vi "NXT Camera Test6.vi"() -> ()   [LabVIEW 2016]
uses:
  <vilib>/NXT/Block Support/NXT_InputPort.ctl
  <vilib>/NXT/Block Support/NXT_OutputPort.ctl
  <vilib>/NXT/NXTIO Xnodes/NXTIONodeSubVIs/NXTMoveMotors.vi
  <vilib>/NXT/NXTIO Xnodes/NXTIONodeSubVIs/NXTStopMotors.vi
  <vilib>/NXT/Dual Mode Library/Waits/Wait_Num.vi
  <vilib>/NXT/Subs/LVHSConnector.ctl
  <vilib>/NXT/NXTIO Xnodes/AddressXNode/NXTIOAddress.xnode
  <vilib>/NXT/NXTIO Xnodes/NXTIOXNode/NXTIO.xnode
  <vilib>/NXT/LegoClasses/BrickReference/BrickReference.lvclass
panel:
  out "Power":bool
  out "X Upper Left":u8
  out "X Lower Right":u8
  out "Y Lower Right":u8
  out "Y Upper Left":u8
  out "Count":u8
  out "Color":u8
  in  "Cluster":T1 {"Tracking Mode" items=["Disable Tracking", "Get First Object", "Get n th Object", "Enable Tracking", "Sort Objects  by size", "Sort Objects  by Colors", "Illumination on ", "Illumination Off", "Write Colormap", "Read Colormap", "Line tracking mode", "Object Tracking mode"]}
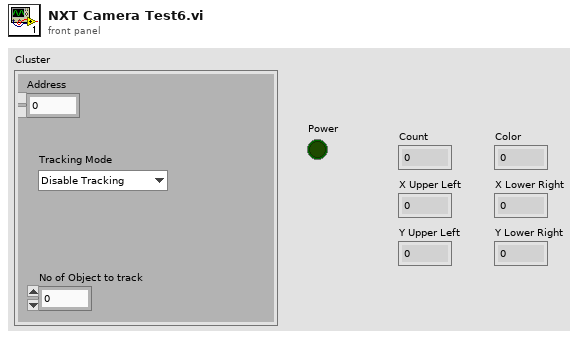
[diagram p1: front panel]
types:
  T1 = cluster{"Address":dbl, "No of Object to track":dbl, "Tracking Mode":u8}
  T2 = cluster{"Tracking Mode":u8, "Object Number to Track":u8, "Address":u8}
  T3 = typedef "NXT_InputPort.ctl" = u32
  T4 = typedef "LVHSConnector.ctl" = refnum<class "BrickReference.lvclass">
  T5 = cluster{"Total Tracked Objects":u8, "Color":u8, "X Upper Left":u8, "Y Upper Left":u8, "X Lower Right":u8, "Y Lower Right":u8, "Status (boolean)":bool}
  T6 = typedef "NXT_OutputPort.ctl" = u8
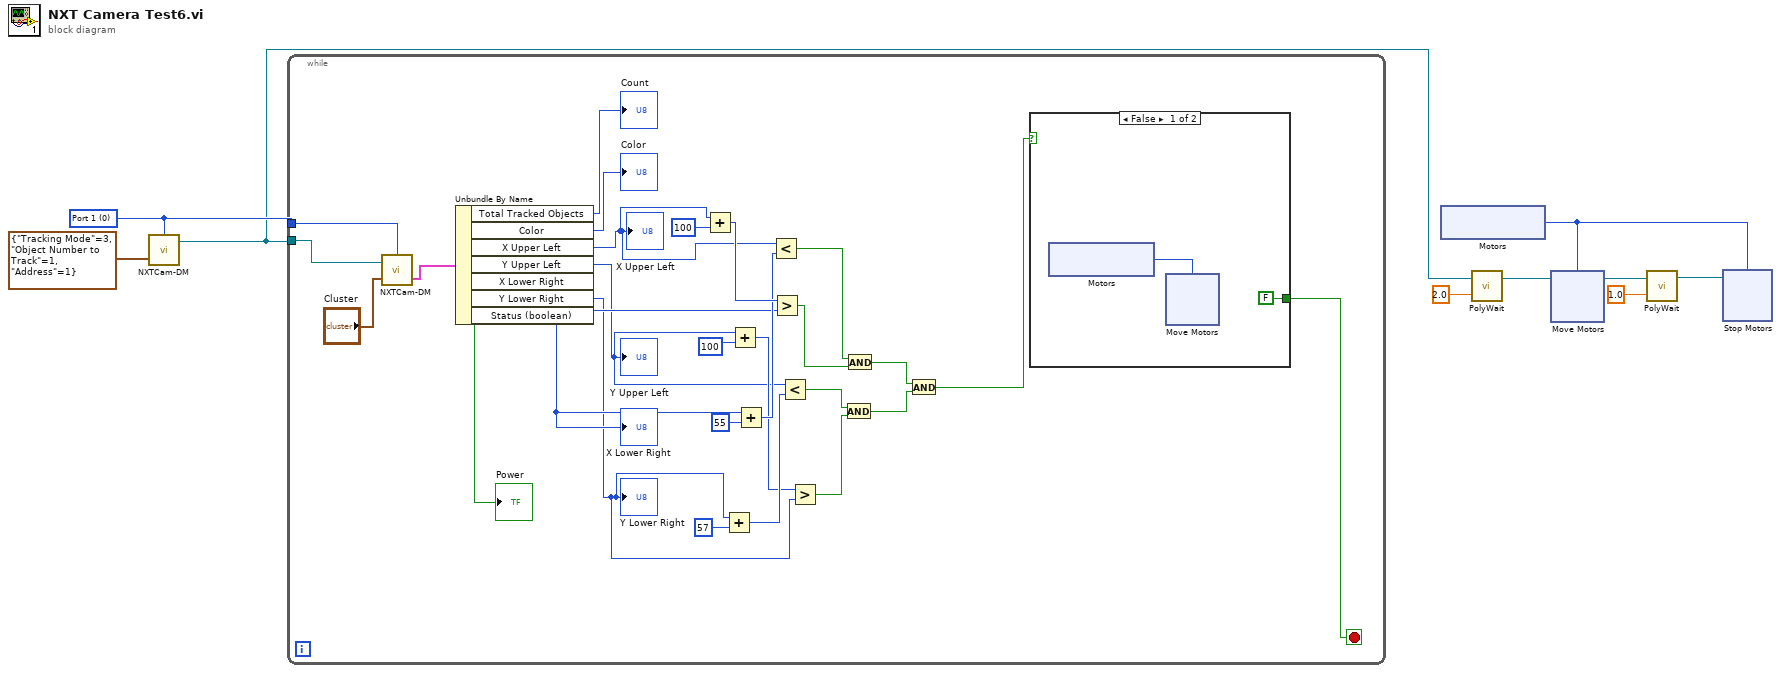
[diagram p0: block diagram]
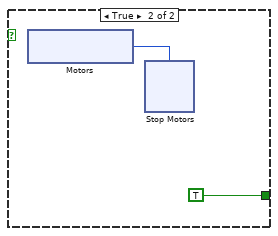
[diagram p2: hidden frame]
diagram:
  w8 = T3 0 items=["Port 1", "Port 2", "Port 3", "Port 4"] ("Input Port")
  n1 = call "NXTCam-DM.vi"("Input of NXTCam"=T2 {"Tracking Mode"=3, "Object Number to Track"=1, "Address"=1}, "Input Port"=w8) -> ("NXT dup"=w7:T4)  [unwired: 1 in, 1 out]
  n2 = while {
    tunnel: w8 -> [w34]
    tunnel: w7 -> [w33]
    stop <- w10 stop-if-true
    n3 = call "NXTCam-DM.vi"("Input of NXTCam"="Cluster", "NXT"=w33, "Input Port"=w34) -> ("Output of NXTCam"=w13:T5)  [unwired: 1 out]
    n4 = Unbundle By Name(w13) -> ("Total Tracked Objects"=→"Count":u8, "Color"=→"Color":u8, "X Upper Left"=w17:u8, "Y Upper Left"=w16:u8, "X Lower Right"=w18:u8, "Y Lower Right"=w15:u8, "Status (boolean)"=→"Power":bool)
    "X Upper Left" <- w17
    "X Lower Right" <- w18
    "Y Lower Right" <- w15
    "Y Upper Left" <- w16
    n5 = Add(x=w17, y=u8 100) -> (x+y=w24:u8)
    n6 = Add(x=w15, y=u8 57) -> (x+y=w27:u8)
    n7 = Add(x=w16, y=u8 100) -> (x+y=w19:u8)
    n8 = Add(x=w18, y=u8 55) -> (x+y=w21:u8)
    n9 = Less?(x=w17, y=w21) -> (x < y?=w22:bool)
    n10 = Greater?(x=w24, y=w18) -> (0:w25:bool)
    n11 = Less?(x=w16, y=w27) -> (x < y?=w28:bool)
    n12 = Greater?(x=w19, y=w15) -> (0:w30:bool)
    n13 = And(x=w28, y=w30) -> (x .and. y?=w32:bool)
    n14 = And(x=w22, y=w25) -> (x .and. y?=w31:bool)
    n15 = And(x=w31, y=w32) -> (x .and. y?=w11:bool)
    n16 = case shown="False" w11 {
      tunnel: [FALSE TRUE] -> w10
      frame False {
        n17 = xnode "Motors"() -> ("Motor"=w38:T6)
        n18 = xnode "Move Motors"("Motors"=w38) -> ()  [unwired: 2 in, 1 out]
      }
      frame True {
        n19 = xnode "Motors"() -> ("Motor"=w48:T6)
        n20 = xnode "Stop Motors"("Motors"=w48) -> ()  [unwired: 1 in, 1 out]
      }
    }
  }
  n21 = xnode "Motors"() -> ("Motor"=w1:T6)
  n22 = call-poly <vilib>:"PolyWait.vi"("Time (1 sec)"=sgl 2.0, "NXT/EV3"=w7) -> ("NXT/EV3"=w5:T4)  [unwired: 2 in]
  n23 = xnode "Move Motors"("Motors"=w1, "NXT/EV3"=w5) -> ("NXT/EV3"=w4:T4)  [unwired: 1 in]
  n24 = call-poly <vilib>:"PolyWait.vi"("Time (1 sec)"=sgl 1.0, "NXT/EV3"=w4) -> ("NXT/EV3"=w2:T4)  [unwired: 2 in]
  n25 = xnode "Stop Motors"("Motors"=w1, "NXT/EV3"=w2) -> ()  [unwired: 1 out]
